vi "ScanTestStart.vi"(7 "VISA resource name":refnum<visa-resource-name>="COM5", 8 "error in (no error)":errorcluster, 9 "Descripbe":string="Start test", 11 "Limit input":string="CH116~1.2~1.6") -> (0 "error out":errorcluster={"status"=TRUE, "code"=-1073807343, "source"="Property Node (arg 1) in VISA Configure Serial Port (Instr).vi->ReadChanel.vi->CheckTestStart.vi"}, 1 "TestData":string="0.000000-----0.000000", 2 "TestResult":bool, 3 "Limit out":string="1.2------1.6", 4 "Descripbe output":string="Start test   (CH116)", 5 "VISA resource name out":refnum<visa-resource-name>)   [LabVIEW 2013]
uses:
  <vilib>/Utility/error.llb/whitespace.ctl
panel:
  in  "Boolean":bool
  # "Waiting Test Start........"
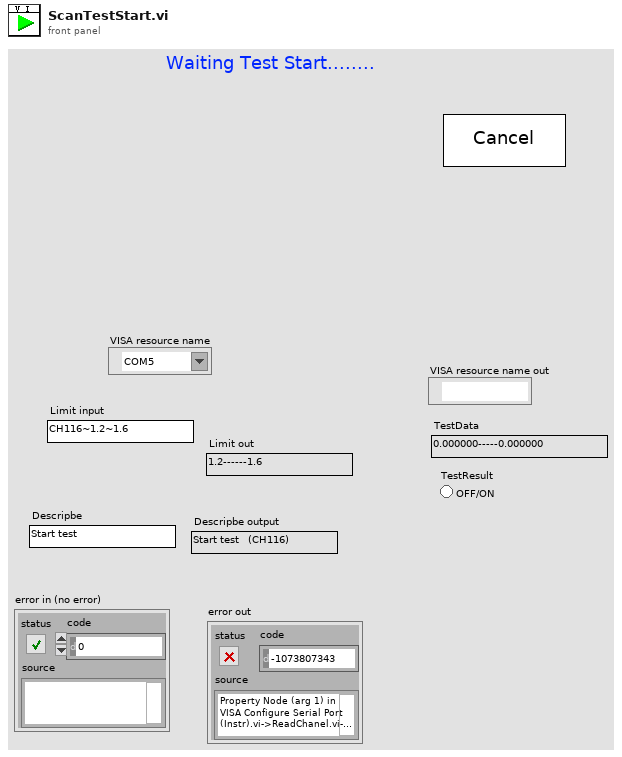
[diagram p1: front panel]
types:
  T1 = typedef "whitespace.ctl" = u16
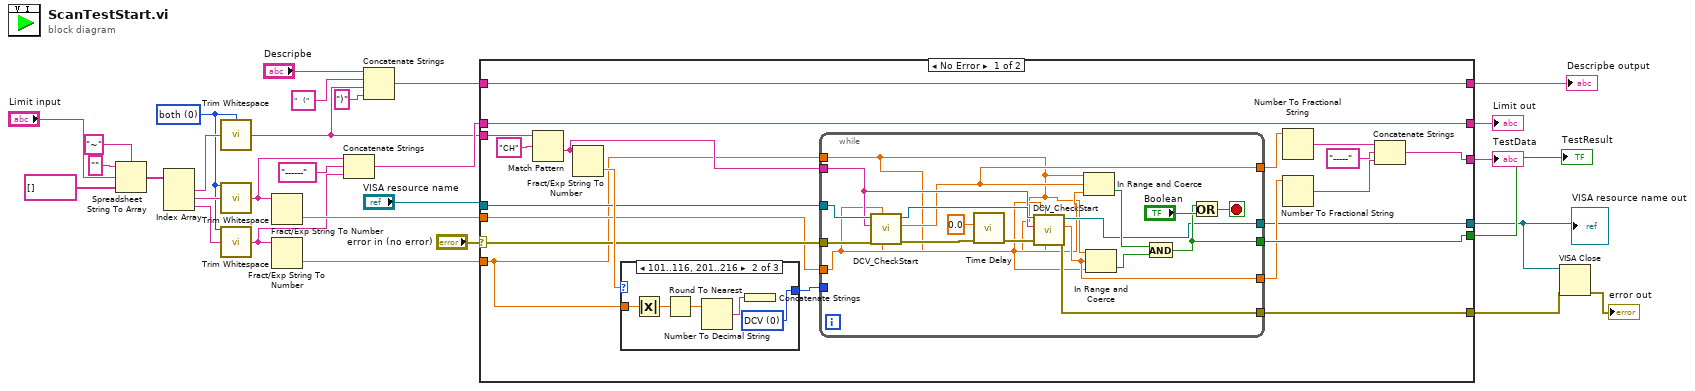
[diagram p0: block diagram]
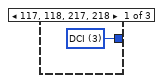
[diagram p2: hidden frame]
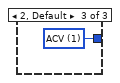
[diagram p3: hidden frame]
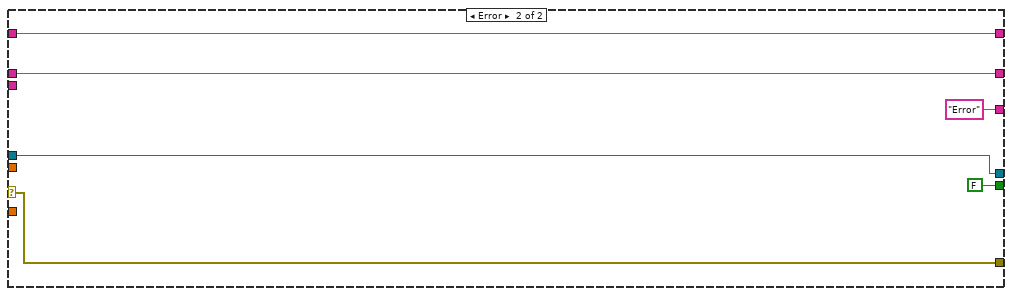
[diagram p4: hidden frame]
diagram:
  w21 = T1 0 items=["both", "start of string", "end of string"] ("location (both)")
  n1 = Spreadsheet String To Array(delimiter (Tab)="~", format string="", spreadsheet string="Limit input", array type (2D Dbl)=string[] []) -> (array=w25:string[])
  n2 = Index Array(array=w25) -> (element #1=w24:string, element #2=w23:string, element #3=w22:string)  [unwired: 3 in]
  n3 = call <vilib>:"Trim Whitespace.vi"("string"=w24, "location (both)"=w21) -> ("trimmed string"=w7:string)
  n4 = call <vilib>:"Trim Whitespace.vi"("string"=w23, "location (both)"=w21) -> ("trimmed string"=w16:string)
  n5 = call <vilib>:"Trim Whitespace.vi"("string"=w22, "location (both)"=w21) -> ("trimmed string"=w15:string)
  n6 = Fract/Exp String To Number(string=w16) -> (number=w20:dbl)  [unwired: 3 in, 1 out]
  n7 = Fract/Exp String To Number(string=w15) -> (number=w18:dbl)  [unwired: 3 in, 1 out]
  n8 = Concatenate Strings(w16, "------" ("string"), w15) -> (w12:string)
  n9 = Concatenate Strings("Descripbe", "   (" ("string"), w7, ")" ("string")) -> (w6:string)
  n10 = case shown="No Error" "error in (no error)" {
    selector: "error in (no error)" -> [w43 w80]
    tunnel: [w30 w80] -> w4
    tunnel: w7 -> [w47 _]
    tunnel: w20 -> [w35 _]
    tunnel: [w41 FALSE] -> w19
    tunnel: w18 -> [w34 _]
    tunnel: "VISA resource name" -> [w42 w75]
    tunnel: [w48 w78] -> w13
    tunnel: w12 -> [w48 w78]
    tunnel: [w46 w77] -> w11
    tunnel: w6 -> [w46 w77]
    tunnel: [w37 "Error" ("read buffer")] -> w5
    tunnel: [w31 w75] -> w1
    frame No Error {
      n11 = Match Pattern(string=w47, regular expression="CH") -> (after substring=w36:string)  [unwired: 1 in, 3 out]
      n12 = Fract/Exp String To Number(string=w36) -> (number=w44:dbl)  [unwired: 3 in, 1 out]
      n13 = case shown="101..116, 201..216" w44 {
        tunnel: w34 -> [_ w73 _]
        tunnel: [w68 w69 w74] -> w45
        frame 117, 118, 217, 218 {
          w68 = u16 3 items=["DCV", "ACV", "AC+DCV", "DCI", "ACI", "AC+DCI", "2Wire Ohms", "4Wire Ohms", "Diode", "Frequency", "Period", "Temperature"] ("Function")
        }
        frame 101..116, 201..216 {
          w69 = u16 0 items=["DCV", "ACV", "AC+DCV", "DCI", "ACI", "AC+DCI", "2Wire Ohms", "4Wire Ohms", "Diode", "Frequency", "Period", "Temperature"] ("Function")
          n14 = Absolute Value(x=w73) -> (abs(x)=w72:dbl)
          n15 = Round To Nearest(number=w72) -> (nearest integer value=w71:dbl)
          n16 = Number To Decimal String(number=w71) -> (decimal integer string=w70:string)  [unwired: 1 in]
          n17 = Concatenate Strings(w70) -> ()  [unwired: 1 out]
        }
        frame 2, Default {
          w74 = u16 1 items=["DCV", "ACV", "AC+DCV", "DCI", "ACI", "AC+DCI", "2Wire Ohms", "4Wire Ohms", "Diode", "Frequency", "Period", "Temperature"] ("Function")
        }
      }
      n18 = while {
        tunnel: w45 -> [_]
        tunnel: w43 -> [w63]
        tunnel: w42 -> [w64]
        tunnel: [w65] -> w41
        tunnel: w36 -> [w58]
        tunnel: w35 -> [w51]
        tunnel: w34 -> [w50]
        tunnel: [w55] -> w33
        tunnel: [w54] -> w32
        tunnel: [w53] -> w31
        tunnel: [w52] -> w30
        stop <- w66 stop-if-true
        n19 = call "DCV_CheckStart.vi"("LowLimit"=w50, "HiLimit"=w51, "Error In"=w63, "channel"=w58, "VISA resource name"=w64) -> ("Error Out"=w62:errorcluster, "value"=w55:dbl, "VISA resource name out"=w59:refnum<visa-resource-name>)  [unwired: 4 in]
        n20 = call "Time Delay"("error in (no error)"=w62, "Delay Time (s)"=0.0) -> ("error out"=w61:errorcluster)  [unwired: 9 in]
        n21 = call "DCV_CheckStart.vi"("LowLimit"=w50, "HiLimit"=w51, "Error In"=w61, "channel"=w58, "VISA resource name"=w59) -> ("Error Out"=w52:errorcluster, "value"=w54:dbl, "VISA resource name out"=w53:refnum<visa-resource-name>)  [unwired: 4 in]
        n22 = In Range and Coerce(upper limit=w50, x=w55, lower limit=w51) -> (In Range?=w56:bool)  [unwired: 1 out]
        n23 = In Range and Coerce(upper limit=w50, x=w54, lower limit=w51) -> (In Range?=w57:bool)  [unwired: 1 out]
        n24 = And(x=w56, y=w57) -> (x .and. y?=w65:bool)
        n25 = Or(x=w65, y="Boolean") -> (x .or. y?=w66:bool)
      }
      n26 = Number To Fractional String(number=w33) -> (F-format string=w40:string)  [unwired: 3 in]
      n27 = Number To Fractional String(number=w32) -> (F-format string=w39:string)  [unwired: 3 in]
      n28 = Concatenate Strings(w40, "-----" ("string"), w39) -> (w37:string)
    }
    frame Error {
    }
  }
  "TestResult" <- w19
  "TestData" <- w5
  "Limit out" <- w13
  "Descripbe output" <- w11
  "VISA resource name out" <- w1
  n29 = VISA Close(VISA resource name=w1, error in (no error)=w4) -> (error out=→"error out":errorcluster)
